vi "Check A_Tunnel on Server.vi"(0 "Values":dbl[](array[numeric]) format="%.2f", 2 "Ch Names":string[](array[string]), 3 "Current Time":dbl format="%.2f", 4 "Adam Loop Count":i32) -> (6 "Scan comment":string)   [LabVIEW 2022 SP3]
uses:
  Anemometry/Anemometry Sub Vis/Controls/In_Range.ctl
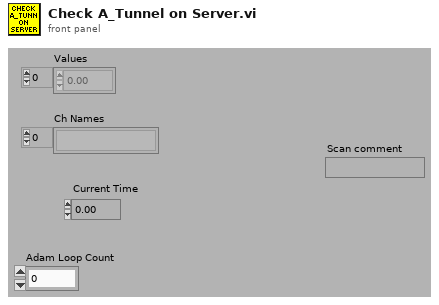
[diagram p1: front panel]
types:
  T1 = typedef "In_Range.ctl" = enum16{"%", "±", "% & ±"}
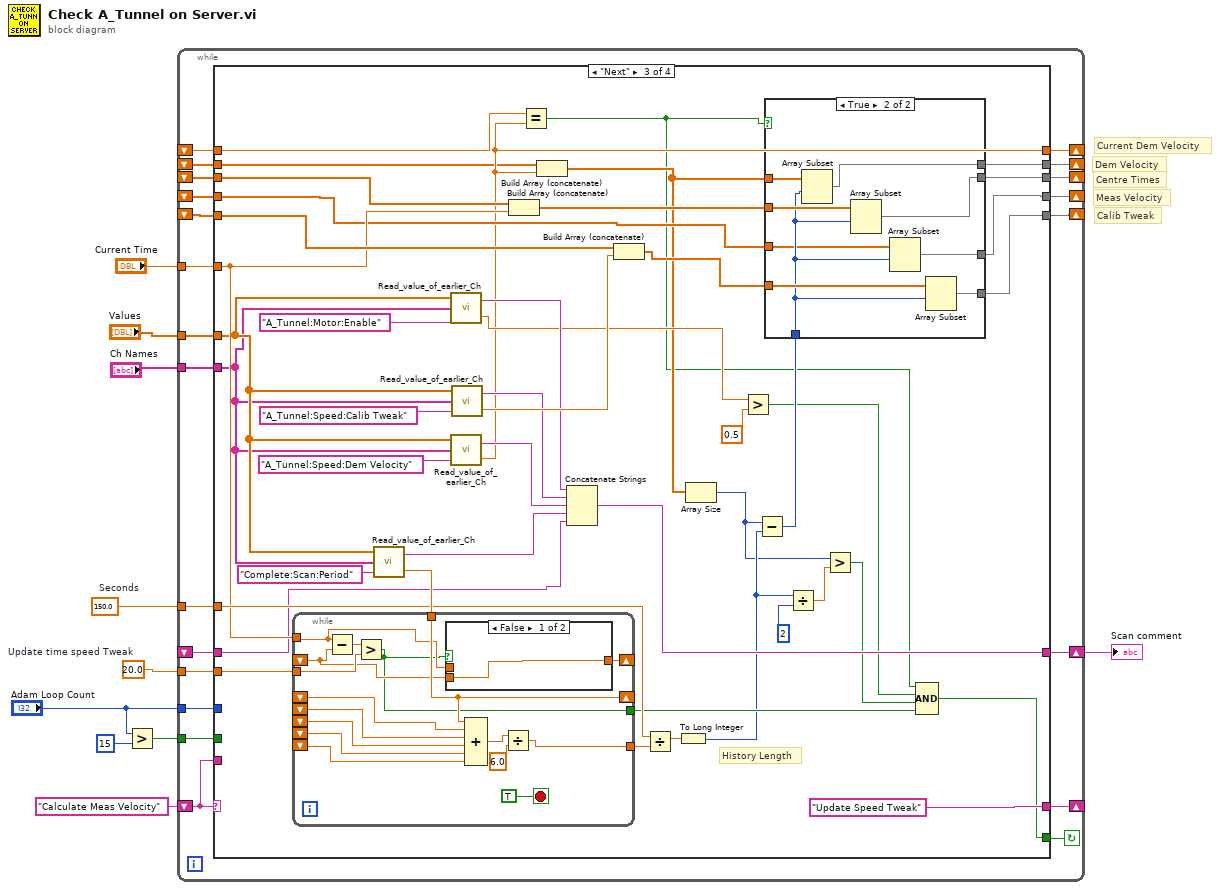
[diagram p0: block diagram]
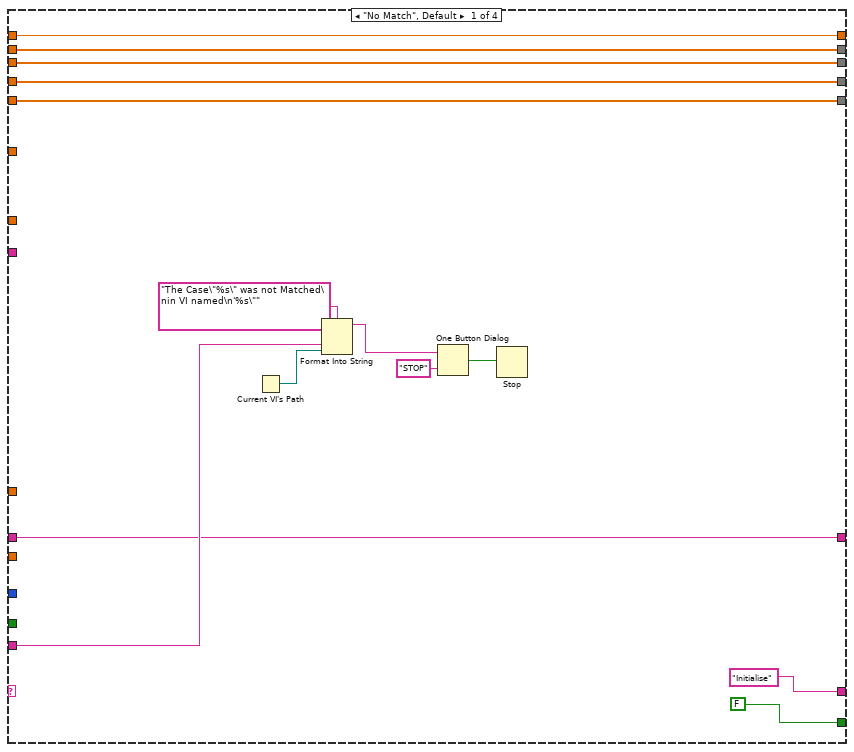
[diagram p2: hidden frame]
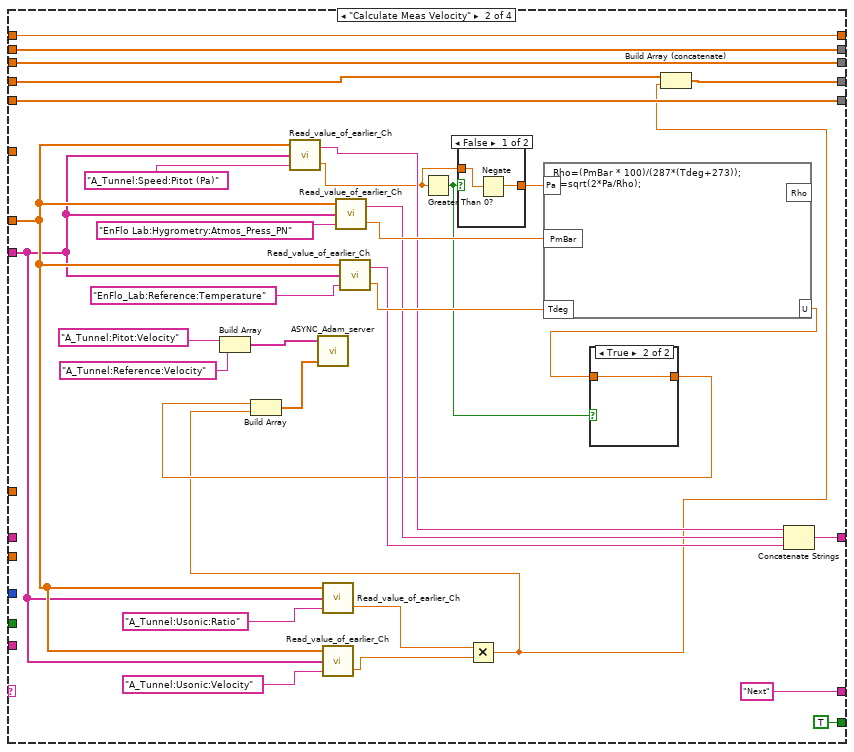
[diagram p3: hidden frame]
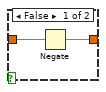
[diagram p4: hidden frame]
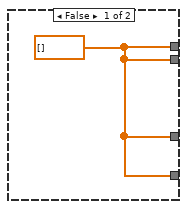
[diagram p6: hidden frame]
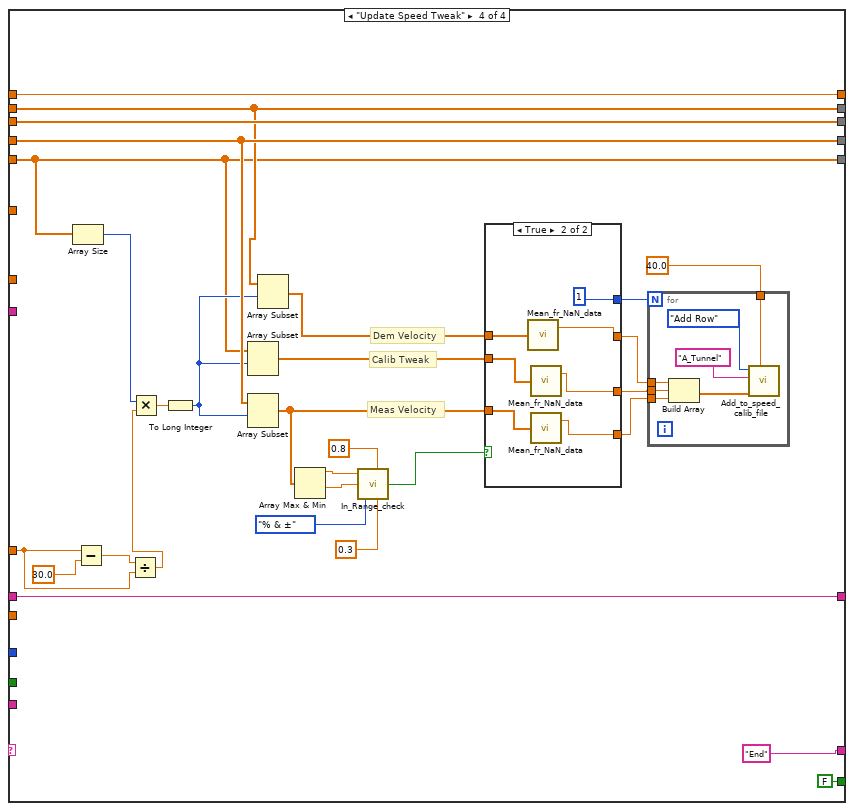
[diagram p8: hidden frame]
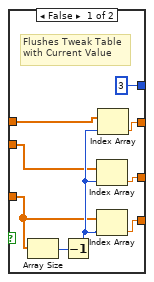
[diagram p9: hidden frame]
diagram:
  w3 = 20.0  # Update time speed Tweak
  w4 = 150.0  # Seconds
  # "Calib Tweak"
  # "Meas Velocity"
  # "Dem Velocity"
  # "Centre Times"
  # "Current Dem Velocity"
  n1 = Greater?(x="Adam Loop Count", y=15) -> (0:w6:bool)
  n2 = while {
    shift-left: "Calculate Meas Velocity" ("t") -> [w30]
    shift-right: [w31] -> _
    tunnel: "Values" -> [w29]
    tunnel: "Ch Names" -> [w28]
    shift-right: [w27] -> _
    shift-left: _ -> [w26]
    shift-right: [w24] -> _
    shift-left: _ -> [w25]
    shift-right: [w21] -> _
    shift-left: _ -> [w22]
    tunnel: "Current Time" -> [w23]
    tunnel: w6 -> [w20]
    shift-right: [w19] -> w5
    shift-left: _ -> [w18]
    tunnel: w4 -> [w17]
    shift-right: [w16] -> _
    shift-left: _ -> [w15]
    shift-right: [w14] -> _
    shift-left: _ -> [w13]
    tunnel: w3 -> [w12]
    tunnel: "Adam Loop Count" -> [w11]
    stop <- w32 continue-if-true
    n3 = case shown="\"Next\"" w30 {
      tunnel: [FALSE TRUE w88 FALSE] -> w32
      tunnel: ["Initialise" "Next" ("t") "Update Speed Tweak" ("t") "End" ("t")] -> w31
      tunnel: w30 -> [w41 _ _ _]
      tunnel: w29 -> [_ w51 w102 _]
      tunnel: w28 -> [_ w50 w101 _]
      tunnel: [w38 w75 w92 w186] -> w27
      tunnel: w26 -> [w38 w75 w89 w186]
      tunnel: w25 -> [w37 w74 w91 w167]
      tunnel: [w37 w74 w126 w167] -> w24
      tunnel: w23 -> [_ _ w112 _]
      tunnel: w22 -> [w36 w73 w125 w185]
      tunnel: [w36 w73 w124 w185] -> w21
      tunnel: w20 -> [_ _ _ _]
      tunnel: [w35 w63 w122 w184] -> w19
      tunnel: w18 -> [w35 _ w95 w184]
      tunnel: w17 -> [_ _ w121 w181]
      tunnel: [w34 w76 w114 w178] -> w16
      tunnel: w15 -> [w34 w78 w96 w178]
      tunnel: [w33 w72 w113 w165] -> w14
      tunnel: w13 -> [w33 w72 w116 w165]
      tunnel: w12 -> [_ _ w111 _]
      tunnel: w11 -> [_ _ _ _]
      frame "No Match", Default {
        n4 = Current VI's Path() -> (path=w40:path)
        n5 = Format Into String(format string="The Case\"%s\" was not Matched\nin VI named\n'%s\"" ("Format String"), w41, w40) -> (resulting string=w44:string)  [unwired: 2 in, 1 out]
        n6 = One Button Dialog(message=w44, button name ("OK")="STOP") -> (true=w42:bool)
        n7 = Stop(stop? (T)=w42) -> ()
      }
      frame "Calculate Meas Velocity" {
        n8 = Build Array("A_Tunnel:Pitot:Velocity", "A_Tunnel:Reference:Velocity") -> (w62:string[])
        n9 = call "Read_value_of_earlier_Ch.vi"("Desired Ch to Read"="A_Tunnel:Speed:Pitot (Pa)", "Ch names"=w50, "Present scan array"=w51) -> ("Value"=w58:dbl, "Scan comment"=w66:string)  [unwired: 1 in]
        n10 = call "Read_value_of_earlier_Ch.vi"("Desired Ch to Read"="A_Tunnel:Usonic:Ratio", "Ch names"=w50, "Present scan array"=w51) -> ("Value"=w49:dbl)  [unwired: 1 in, 1 out]
        n11 = call "Read_value_of_earlier_Ch.vi"("Desired Ch to Read"="A_Tunnel:Usonic:Velocity", "Ch names"=w50, "Present scan array"=w51) -> ("Value"=w48:dbl)  [unwired: 1 in, 1 out]
        n12 = call "Read_value_of_earlier_Ch.vi"("Desired Ch to Read"="EnFlo Lab:Hygrometry:Atmos_Press_PN", "Ch names"=w50, "Present scan array"=w51) -> ("Value"=w68:dbl, "Scan comment"=w65:string)  [unwired: 1 in]
        n13 = call "Read_value_of_earlier_Ch.vi"("Desired Ch to Read"="EnFlo_Lab:Reference:Temperature", "Ch names"=w50, "Present scan array"=w51) -> ("Value"=w67:dbl, "Scan comment"=w64:string)  [unwired: 1 in]
        n14 = Greater Than 0?(x=w58) -> (x > 0?=w57:bool)
        n15 = case shown="False" w57 {
          tunnel: [w83 w85] -> w59
          tunnel: w58 -> [w84 w85]
          frame False {
            n16 = Negate(x=w84) -> (-x=w83:dbl)
          }
          frame True {
          }
        }
        n17 = Multiply(x=w49, y=w48) -> (x*y=w47:dbl)
        n18 = formula code="Rho=(PmBar * 100)/(287*(Tdeg+273));\nU=sqrt(2*Pa/Rho);"("Pa"=w59, "Tdeg"=w67, "PmBar"=w68) -> ("U"=w56:dbl)  [unwired: 1 out]
        n19 = case shown="True" w57 {
          tunnel: w56 -> [w81 w82]
          tunnel: [w80 w82] -> w55
          frame False {
            n20 = Negate(x=w81) -> (-x=w80:dbl)
          }
          frame True {
          }
        }
        n21 = Build Array(w55, w47) -> (w61:dbl[])
        n22 = call "ASYNC_Adam_server.vi"("Values"=w61, "Channel Names"=w62) -> ()  [unwired: 1 in, 3 out]
        n23 = Build Array (concatenate)(w78, w47) -> (w76:dbl[])
        n24 = Concatenate Strings(w66, w65, w64) -> (w63:string)
      }
      frame "Next" {
        # "History Length"
        n25 = call "Read_value_of_earlier_Ch.vi"("Desired Ch to Read"="Complete:Scan:Period", "Ch names"=w101, "Present scan array"=w102) -> ("Value"=w129:dbl, "Scan comment"=w123:string)  [unwired: 1 in]
        n26 = while {
          shift-right: [w156] -> _
          shift-left: _ -> [w155]
          tunnel: w129 -> [w156]
          shift-left: _ -> [w154]
          shift-left: _ -> [w153]
          shift-left: _ -> [w152]
          shift-left: _ -> [w151]
          tunnel: [w147] -> w128
          tunnel: w112 -> [w143]
          shift-right: [w144] -> _
          shift-left: _ -> [w142]
          tunnel: w111 -> [w145]
          tunnel: [w141] -> w110
          stop <- TRUE stop-if-true
          n27 = Subtract(x=w143, y=w142) -> (x-y=w146:dbl)
          n28 = Greater?(x=w146, y=w145) -> (0:w141:bool)
          n29 = case shown="False" w141 {
            tunnel: [w157 w158] -> w144
            tunnel: w143 -> [_ w158]
            tunnel: w142 -> [w157 _]
            frame False {
            }
            frame True {
            }
          }
          n30 = Compound Arithmetic op=ADD(w156, w155, w154, w153, w152, w151) -> (w149:dbl)
          n31 = Divide(x=w149, y=6.0) -> (x/y=w147:dbl)
        }
        n32 = call "Read_value_of_earlier_Ch.vi"("Desired Ch to Read"="A_Tunnel:Motor:Enable", "Ch names"=w101, "Present scan array"=w102) -> ("Value"=w98:dbl, "Scan comment"=w99:string)  [unwired: 1 in]
        n33 = call "Read_value_of_earlier_Ch.vi"("Desired Ch to Read"="A_Tunnel:Speed:Dem Velocity", "Ch names"=w101, "Present scan array"=w102) -> ("Value"=w92:dbl, "Scan comment"=w108:string)  [unwired: 1 in]
        n34 = call "Read_value_of_earlier_Ch.vi"("Desired Ch to Read"="A_Tunnel:Speed:Calib Tweak", "Ch names"=w101, "Present scan array"=w102) -> ("Value"=w117:dbl, "Scan comment"=w109:string)  [unwired: 1 in]
        n35 = Build Array (concatenate)(w125, w112) -> (w118:dbl[])
        n36 = Equal?(x=w89, y=w92) -> (x = y?=w87:bool)
        n37 = Build Array (concatenate)(w91, w92) -> (w90:dbl[])
        n38 = Concatenate Strings(w99, w109, w108, w123, w95) -> (w122:string)
        n39 = Build Array (concatenate)(w116, w117) -> (w115:dbl[])
        n40 = Divide(x=w121, y=w128) -> (x/y=w127:dbl)
        n41 = To Long Integer(number=w127) -> (32bit integer=w106:i32)
        n42 = Array Size(array=w90) -> (size(s)=w86:i32)
        n43 = Greater?(x=w98, y=0.5) -> (0:w94:bool)
        n44 = Subtract(x=w86, y=w106) -> (x-y=w103:i32)
        n45 = case shown="True" w87 {
          tunnel: [w131 w140] -> w126
          tunnel: w90 -> [_ w139]
          tunnel: [w131 w138] -> w124
          tunnel: w118 -> [_ w137]
          tunnel: w115 -> [_ w136]
          tunnel: [w131 w135] -> w114
          tunnel: [w131 w134] -> w113
          tunnel: w103 -> [_ w133]
          tunnel: w96 -> [_ w132]
          frame False {
            w131 = dbl[] []
          }
          frame True {
            n46 = Array Subset(array=w139, index=w133) -> (w140:dbl[])  [unwired: 1 in]
            n47 = Array Subset(array=w137, index=w133) -> (w138:dbl[])  [unwired: 1 in]
            n48 = Array Subset(array=w132, index=w133) -> (w135:dbl[])  [unwired: 1 in]
            n49 = Array Subset(array=w136, index=w133) -> (w134:dbl[])  [unwired: 1 in]
          }
        }
        n50 = Divide(x=w106, y=2) -> (x/y=w105:dbl)
        n51 = Greater?(x=w86, y=w105) -> (0:w104:bool)
        n52 = Compound Arithmetic op=AND(w87, w94, w104, w110) -> (w88:bool)
      }
      frame "Update Speed Tweak" {
        # "Meas Velocity"
        # "Calib Tweak"
        # "Dem Velocity"
        n53 = Array Size(array=w165) -> (size(s)=w164:i32)
        n54 = Subtract(x=w181, y=30.0) -> (x-y=w182:dbl)
        n55 = Divide(x=w182, y=w181) -> (x/y=w180:dbl)
        n56 = Multiply(x=w164, y=w180) -> (x*y=w179:dbl)
        n57 = To Long Integer(number=w179) -> (32bit integer=w177:i32)
        n58 = Array Subset(array=w165, index=w177) -> (w175:dbl[])  [unwired: 1 in]
        n59 = Array Subset(array=w178, index=w177) -> (w174:dbl[])  [unwired: 1 in]
        n60 = Array Subset(array=w167, index=w177) -> (w176:dbl[])  [unwired: 1 in]
        n61 = Array Max & Min(array=w174) -> (max value=w173:dbl, min value=w172:dbl)  [unwired: 2 out]
        n62 = call "In_Range_check.vi"("±"=0.3, "%"=0.8, "Mode"=In_Range."% & ±", "Value"=w172, "Setpoint"=w173) -> ("In Range"=w168:bool)  [unwired: 2 out]
        n63 = case shown="True" w168 {
          tunnel: w176 -> [w201 w210]
          tunnel: w175 -> [w200 w209]
          tunnel: w174 -> [w199 w208]
          tunnel: [w198 w207] -> w163
          tunnel: [w197 w206] -> w162
          tunnel: [w196 w205] -> w161
          tunnel: [3 1] -> w160
          frame False {
            # "Flushes Tweak Table\nwith Current Value"
            n64 = Array Size(array=w199) -> (size(s)=w203:i32)
            n65 = Decrement(x=w203) -> (x-1=w202:i32)
            n66 = Index Array(array=w200, index=w202) -> (element=w197:dbl)
            n67 = Index Array(array=w199, index=w202) -> (element=w198:dbl)
            n68 = Index Array(array=w201, index=w202) -> (element=w196:dbl)
          }
          frame True {
            n69 = call "Mean_fr_NaN_data.vi"("Data"=w210) -> ("Mean value"=w205:dbl)  [unwired: 1 out]
            n70 = call "Mean_fr_NaN_data.vi"("Data"=w209) -> ("Mean value"=w206:dbl)  [unwired: 1 out]
            n71 = call "Mean_fr_NaN_data.vi"("Data"=w208) -> ("Mean value"=w207:dbl)  [unwired: 1 out]
          }
        }
        n72 = for {
          N: w160 -> [_]
          tunnel: w163 -> [w191]
          tunnel: w162 -> [w190]
          tunnel: w161 -> [w189]
          tunnel: 40.0 ("Max Velocity") -> [w188]
          n73 = Build Array(w189, w190, w191) -> (w192:dbl[])
          n74 = call "Add_to_speed_calib_file.vi"("Max Velocity"=w188, "New Row"=w192, "Rig Name"="A_Tunnel" ("y"), "Mode"=enum16{"Add Row", "Get Error Value"}."Add Row") -> ()  [unwired: 2 in, 2 out]
        }
      }
    }
  }
  "Scan comment" <- w5
